vi "Emballage_BDD_choix_Config_Filtre.vi"(8 "Error in":errorcluster caption="Error in (no error)", 10 "where valeur":string[](array[string]), 11 "Where colonne":string[](array[string])) -> (0 "Error out":errorcluster)   [LabVIEW 2020]
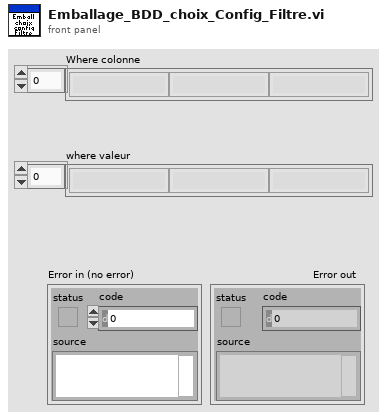
[diagram p1: front panel]
types:
  T1 = typedef "Choix_Config_ref.ctl" = cluster{"No_Valve_FAS":refnum<vi>, "Liste multicolonne":refnum<vi>, "suffixe":refnum<vi>, "designation":refnum<vi>, "Famille":refnum<vi>}
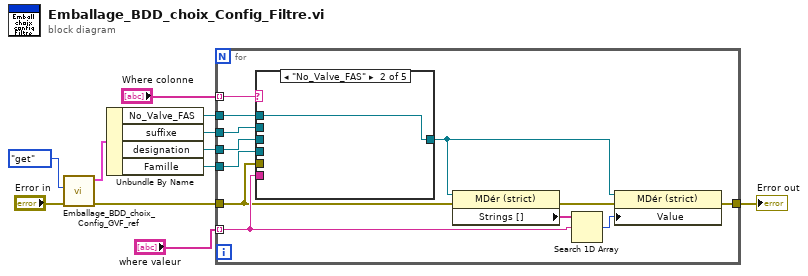
[diagram p0: block diagram]
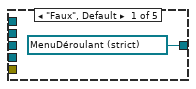
[diagram p2: hidden frame]
diagram:
  n1 = call "Emballage_BDD_choix_Config_GVF_ref.vi"("Error in"="Error in", "Énum"=enum16{"get", "set"}."get") -> ("Error out"=w5:errorcluster, "Cluster OUT"=w10:T1)  [unwired: 8 in]
  n2 = Unbundle By Name(w10) -> ("No_Valve_FAS"=w6:refnum<vi>, "suffixe"=w3:refnum<vi>, "designation"=w2:refnum<vi>, "Famille"=w1:refnum<vi>)
  n3 = for {
    tunnel: "where valeur" -> [w21] mode=indexing
    tunnel: "Where colonne" -> [w22] mode=indexing
    tunnel: w6 -> [w23]
    tunnel: w5 -> [w20]
    tunnel: [w16] -> w4
    tunnel: w3 -> [w15]
    tunnel: w2 -> [w14]
    tunnel: w1 -> [w13]
    n4 = case shown="\"No_Valve_FAS\"" w22 {
      tunnel: [refnum<vi> refnum ("Famille") w25 w26 w27 w28] -> w12
      tunnel: w23 -> [_ w25 _ _ _]
      tunnel: w21 -> [_ _ _ _ _]
      tunnel: w20 -> [_ _ _ _ _]
      tunnel: w15 -> [_ _ w26 _ _]
      tunnel: w14 -> [_ _ _ w27 _]
      tunnel: w13 -> [_ _ _ _ w28]
      frame "Faux", Default {
      }
      frame "No_Valve_FAS" {
      }
      frame "suffixe" {
      }
      frame "designation" {
      }
      frame "Famille" {
      }
    }
    n5 = property class="MDér (strict)"(reference=w12, error in=w20) -> (error out=w17:errorcluster, "Strings []"=w19:string[])  [unwired: 1 out]
    n6 = Search 1D Array(1D array=w19, element=w21) -> (index of element=w18:i32)  [unwired: 1 in]
    n7 = property class="MDér (strict)"(reference=w12, error in=w17, "Value"=w18) -> (error out=w16:errorcluster)  [unwired: 1 out]
  }
  "Error out" <- w4
